vi "Handle Error.vi"(8 "error in (no error)":errorcluster, 11 "Controller in":refnum<class "Controller.lvclass">) -> (0 "error out":errorcluster, 2 "stop actor?":bool=TRUE, 3 "Controller out":refnum<class "Controller.lvclass">)   [LabVIEW 2016, in "Controller Actor.lvlib" / "Controller.lvclass"]
doc: "(<B>Filename</B>: Actor Framework.lvlib:Actor.lvclass:Handle Error.vi)\n\nDefines how the actor handles an error that occurred while processing a message.\n\nBy default, this method does nothing except stop the actor. This method also treats error code 43 (coming from <B>error in</B>) as a sign that the actor shut down normally. In this situation, the Handle Error method does not return the error on <B>error out</B>, meaning the actor's caller will not receive it. All other error codes will be returned on <B>error out</B>.\n\nA descendant class may override this method to change this behavior."
uses:
  <userlib>/Common Components/Controller/Controller.lvclass
  <vilib>/ActorFramework/Actor/Actor.lvclass
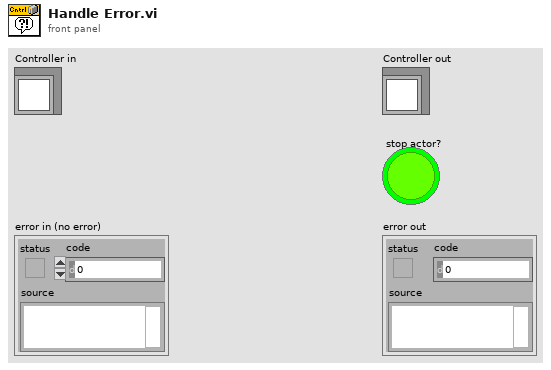
[diagram p1: front panel]
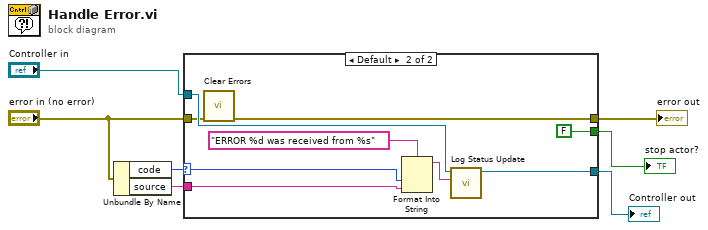
[diagram p0: block diagram]
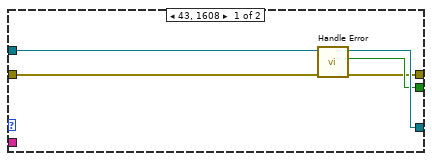
[diagram p2: hidden frame]
diagram:
  n1 = Unbundle By Name("error in (no error)") -> ("code"=w3:i32, "source"=w4:string)
  n2 = case shown="Default" w3 {
    selector: w3 -> [_ w14]
    tunnel: "Controller in" -> [w11 w21]
    tunnel: [w12 w20] -> w7
    tunnel: "error in (no error)" -> [w9 w19]
    tunnel: [w8 w18] -> w6
    tunnel: [w10 FALSE ("stop actor?")] -> w5
    tunnel: w4 -> [_ w15]
    frame 43, 1608 {
      n3 = call-parent "Handle Error.vi"("error in (no error)"=w9, "Actor in"=w11) -> ("error out"=w8:errorcluster, "stop actor?"=w10:bool, "Actor out"=w12:refnum<class "Controller.lvclass">)  [unwired: 7 in]
    }
    frame Default {
      n4 = call <vilib>:"Clear Errors.vi"("error in (no error)"=w19) -> ("error out"=w18:errorcluster)  [unwired: 5 in, 1 out]
      n5 = Format Into String(format string="ERROR %d was received from %s", w14, w15) -> (resulting string=w13:string)  [unwired: 2 in, 1 out]
      n6 = call-dynamic "Log Status Update.vi"("String"=w13, "Controller in"=w21) -> ("Controller out"=w20:refnum<class "Controller.lvclass">)  [unwired: 8 in, 1 out]
    }
  }
  "Controller out" <- w7
  "error out" <- w6
  "stop actor?" <- w5
